vi "acquisition_son.vi"(8 "entrée d'erreur (pas d'erreur)":errorcluster, 10 "ID de tâche":T1 format="%.0x", 11 "file d'attente":refnum<queue>) -> (0 "sortie d'erreur":errorcluster, 2 "ID de tâche en sortie":T1 format="%.0x", 3 "file d'attente en sortie":refnum<queue>)   [LabVIEW 2017]
doc: "Bloc qui gére l'acquisition du son (environ 100ms par acquisition)"
uses:
  <vilib>/sound2/lvsound2.llb/Sound Input Task ID.ctl
  variable_stop_globale.vi
  <vilib>/sound2/lvsound2.llb/Sound Input Read (DBL).vi
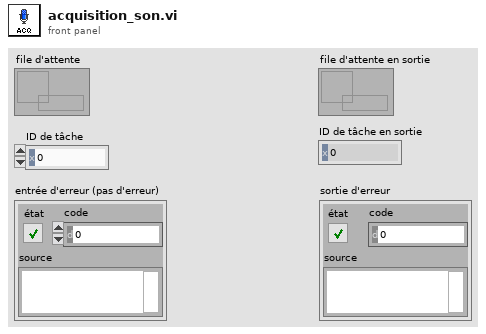
[diagram p1: front panel]
types:
  T1 = typedef "Sound Input Task ID.ctl" = u32
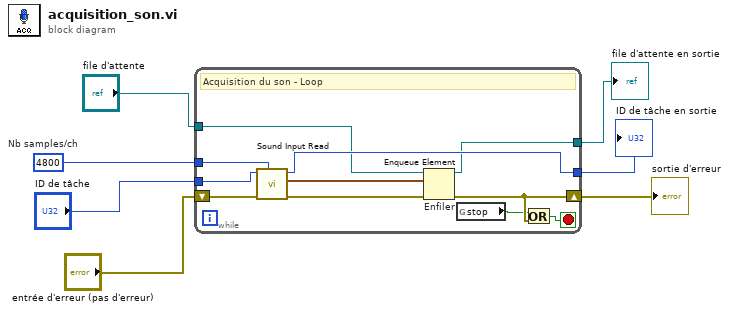
[diagram p0: block diagram]
diagram:
  w1 = 4800  # Nb samples/ch
  n1 = while "Entrée" {
    shift-right: [w12] -> w7
    shift-left: "entrée d'erreur (pas d'erreur)" -> [w18]
    tunnel: [w16] -> w6
    tunnel: "file d'attente" -> [w15]
    tunnel: [w13] -> w2
    tunnel: w1 -> [w11]
    tunnel: "ID de tâche" -> [w10]
    stop <- w8 stop-if-true
    # "Acquisition du son - Loop"
    n2 = call-poly <vilib>:"Sound Input Read.vi"("number of samples/ch"=w11, "error in (no error)"=w18, "task ID"=w10) -> ("error out"=w14:errorcluster, "data"=w17:waveform(dbl)[], "task ID out"=w16:T1)  [unwired: 6 in]
    n3 = Enqueue Element "Enfiler"(queue=w15, element=w17, error in (no error)=w14) -> (queue out=w13:refnum<queue>, error out=w12:errorcluster)  [unwired: 1 in, 1 out]
    n4 = global read "variable_stop_globale.vi" "stop"() -> (w9:bool)
    n5 = Or(x=w9, y=w12) -> (x .or. y?=w8:bool)
  }
  "ID de tâche en sortie" <- w6
  "sortie d'erreur" <- w7
  "file d'attente en sortie" <- w2
